vi "Part 2.vi"() -> ()   [LabVIEW 2021]
uses:
  <userlib>/_OpenG.lib/string/string.llb/Convert EOLs (String)__ogtk.vi
  <vilib>/Analysis/NI_AAL_Geometry.lvlib
  <vilib>/Analysis/NI_AALBase.lvlib
  <resource>/lvanlys.dll
  <vilib>/Analysis/baseanly.llb/Real Dot Product.vi
panel:
  out "size(s)":i32=6405262
  in  "Input":string="R 9 (#521d52)\nU 5 (#11e893)\nR 4 (#079312)\nU 4 (#5458e3)\nR 7 (#233422)\nU 3 (#664171)\nL 3 (#475012)\nU 6 (#312e21)\nR 6 (#024a22)\nU 3 (#335f61)\nL 6 (#699da2)\nU 4 (#3d7d41)\nL 6 (#699da0)\nU 7 (#125e51)\nL 3 (#1861e2)\nD 7 (#09f8e1)\nL 4 (#70eb32)\nD 10 (#31c8a3)\nR 4 (#0685e2)\nD 3 (#247e93)\nL 8 (#260972)\nU 7 (#36eca3)\nL 8 (#40b8d2)\nU 5 (#312e23)\nL 7 (#3c4242)\nU 8 (#50c7a3)\nR 6 (#21b062)\nU 7 (#443963)\nL 6 (#0f6920)\nU 5 (#2e1d73)\nL 3 (#6f8330)\nD 3 (#1a4943)\nL 5 (#5cebe2)\nD 12 (#27c9f3)\nR 5 (#220072)\nD 3 (#5adb73)\nL 6 (#317f72)\nD 2 (#053831)\nL 7 (#0c0802)\nU 5 (#124b51)\nL 5 (#198d90)\nD 11 (#46f3b1)\nL 5 (#198d92)\nD 2 (#5424f1)\nL 3 (#1232f2)\nU 4 (#408801)\nL 6 (#18cc52)\nU 4 (#3a6ed1)\nR 6 (#38c312)\nU 5 (#299193)\nL 3 (#2c9e72)\nU 3 (#5c2593)\nR 3 (#2cf822)\nU 5 (#33d851)\nR 4 (#1b0740)\nU 2 (#109221)\nR 9 (#1b0742)\nU 4 (#414cb1)\nL 7 (#0838d2)\nU 5 (#1ea173)\nL 2 (#3fcef2)\nU 7 (#3502f3)\nL 3 (#6d0672)\nU 3 (#0ea733)\nL 4 (#2c94c2)\nU 12 (#4ec103)\nL 4 (#041640)\nD 3 (#4bae23)\nL 3 (#4ff660)\nD 9 (#4bae21)\nL 4 (#458e90)\nD 7 (#202933)\nL 3 (#3fcef0)\nD 6 (#4b45b3)\nR 7 (#710a62)\nD 4 (#111783)\nR 4 (#264f12)\nD 4 (#19e183)\nL 5 (#361fa2)\nD 7 (#19e181)\nL 6 (#27a082)\nD 6 (#188573)\nL 7 (#187f60)\nU 8 (#343903)\nL 4 (#4719a0)\nU 4 (#1abc03)\nL 4 (#0e8d22)\nU 8 (#31faf3)\nL 3 (#7a8270)\nD 12 (#21cf23)\nL 4 (#7a8272)\nD 12 (#2cc503)\nR 4 (#0e8d20)\nD 5 (#0623c3)\nL 9 (#42cc80)\nU 3 (#320273)\nL 2 (#372482)\nU 5 (#11b943)\nL 7 (#10cb12)\nU 10 (#11b941)\nL 2 (#41f692)\nU 5 (#20ece3)\nL 5 (#13b450)\nU 6 (#367f33)\nL 3 (#2a3b50)\nD 9 (#1c7473)\nL 4 (#461d20)\nD 9 (#52f3a1)\nR 4 (#0bc750)\nD 5 (#208061)\nL 6 (#34c310)\nD 2 (#058993)\nL 5 (#0a5680)\nD 6 (#0a6a63)\nL 10 (#1056f0)\nD 2 (#47eba3)\nL 5 (#1056f2)\nD 3 (#3bd443)\nL 7 (#20ad20)\nD 9 (#05bb21)\nL 2 (#1efac0)\nD 7 (#770991)\nL 7 (#429760)\nD 11 (#16ef21)\nL 2 (#365170)\nU 11 (#208063)\nL 8 (#77b350)\nU 6 (#4828a3)\nL 5 (#023210)\nU 5 (#23f413)\nL 3 (#45da92)\nU 4 (#3712a3)\nR 6 (#45da90)\nD 5 (#4805f3)\nR 3 (#1d94d0)\nU 5 (#135023)\nR 5 (#12ee60)\nU 7 (#1ed111)\nL 4 (#1b3730)\nU 11 (#6b41c1)\nL 5 (#3ecd30)\nD 11 (#27e453)\nL 5 (#0e45d2)\nU 3 (#35a2b3)\nL 3 (#0e45d0)\nD 6 (#2c8bd3)\nL 3 (#510880)\nD 8 (#5860e3)\nL 5 (#318662)\nU 5 (#755013)\nL 3 (#318660)\nU 8 (#6ac523)\nL 3 (#233450)\nU 3 (#6aa731)\nL 4 (#498890)\nU 11 (#6aa733)\nR 2 (#46f1c0)\nU 10 (#41ea11)\nR 8 (#22c9f2)\nU 6 (#3198b1)\nR 6 (#7541d0)\nU 7 (#28ad81)\nR 6 (#7541d2)\nD 5 (#295961)\nR 9 (#22c9f0)\nU 5 (#396ab1)\nR 4 (#32ead0)\nU 8 (#4cd1e1)\nR 7 (#372ca0)\nU 5 (#192443)\nL 7 (#0df120)\nU 9 (#3417c3)\nL 5 (#2818d0)\nU 4 (#421ca1)\nR 6 (#444470)\nU 5 (#421ca3)\nL 9 (#147140)\nU 5 (#2c7e73)\nR 9 (#2c5cf0)\nU 3 (#6b8981)\nR 6 (#216860)\nU 6 (#37e4d1)\nR 4 (#10dd20)\nU 8 (#0f9fe1)\nR 3 (#596772)\nU 3 (#52ae11)\nR 7 (#596770)\nU 5 (#1cee91)\nR 4 (#3b6fc0)\nU 7 (#1dcb51)\nL 3 (#2360d0)\nU 4 (#643831)\nL 12 (#4537b0)\nU 4 (#180df1)\nR 9 (#31cd00)\nU 7 (#23f461)\nR 6 (#609520)\nU 7 (#10d611)\nR 3 (#2b2910)\nD 12 (#150921)\nR 5 (#45e700)\nD 5 (#4e7701)\nR 5 (#1eaa20)\nU 7 (#43e531)\nR 9 (#0f10f0)\nU 3 (#29c2d1)\nR 8 (#6ca0d0)\nU 10 (#28c611)\nR 3 (#19ef80)\nD 5 (#4d5381)\nR 9 (#30dd00)\nD 2 (#4c2151)\nR 4 (#480fe0)\nD 5 (#4bdcd1)\nR 4 (#4cc442)\nD 2 (#1122d1)\nR 3 (#08cce2)\nD 6 (#5309a1)\nR 4 (#1118f0)\nD 3 (#1e9b31)\nR 4 (#447830)\nD 10 (#0b6561)\nR 4 (#246dd0)\nD 7 (#5ca761)\nR 5 (#356150)\nD 4 (#09fb01)\nR 6 (#3786e2)\nD 7 (#5f9be1)\nR 7 (#42ca92)\nU 5 (#019611)\nR 8 (#1005b2)\nU 3 (#21ae81)\nR 6 (#173bf2)\nU 4 (#49b611)\nR 3 (#2022c0)\nU 6 (#33a5e1)\nR 8 (#3040d0)\nU 9 (#34b873)\nL 3 (#4a8800)\nU 2 (#34b871)\nL 5 (#06a780)\nU 5 (#08d321)\nL 4 (#4c2b40)\nU 6 (#696b43)\nL 4 (#1ca7c0)\nD 9 (#454c43)\nL 2 (#1f13f0)\nD 2 (#078593)\nL 7 (#1135a0)\nU 9 (#0641a3)\nR 3 (#0bf850)\nU 10 (#6b57e3)\nR 3 (#2d9de2)\nU 4 (#5f4661)\nR 7 (#33d1f2)\nU 6 (#5f4663)\nR 5 (#5a9aa2)\nU 6 (#4fc703)\nR 2 (#4f6cf0)\nU 2 (#0b8203)\nR 11 (#3efc40)\nU 5 (#0b8201)\nR 12 (#2da140)\nU 7 (#20f823)\nR 2 (#380710)\nU 6 (#339af3)\nR 3 (#514cf0)\nD 11 (#087ee3)\nR 7 (#4ad610)\nU 11 (#0e30f1)\nR 7 (#1235d2)\nU 9 (#60a251)\nL 6 (#3c6422)\nU 5 (#60a253)\nL 8 (#33f7d2)\nD 6 (#35e7b1)\nL 6 (#511ed2)\nU 6 (#087321)\nL 5 (#2e2a40)\nU 6 (#38d611)\nR 7 (#233f70)\nU 4 (#143ab1)\nL 10 (#05c470)\nU 4 (#007f61)\nL 5 (#189c70)\nU 4 (#633781)\nR 6 (#568f40)\nU 4 (#258a01)\nR 4 (#0d56c0)\nD 4 (#4866e1)\nR 5 (#4b3420)\nU 3 (#060511)\nR 5 (#100980)\nD 10 (#636631)\nR 2 (#230f20)\nD 3 (#1720b1)\nR 4 (#160300)\nD 2 (#3075f3)\nR 4 (#773320)\nU 2 (#370a93)\nR 3 (#6201c0)\nU 11 (#130763)\nR 8 (#24c420)\nD 9 (#130761)\nR 4 (#4767f0)\nD 4 (#49bd53)\nR 5 (#183ae2)\nD 6 (#36b133)\nL 5 (#6b61f2)\nD 7 (#36b131)\nL 4 (#2a6482)\nD 7 (#4570b3)\nR 6 (#202c82)\nD 4 (#30c3c3)\nR 7 (#2fc410)\nD 8 (#11c203)\nL 8 (#320302)\nD 6 (#1b7b81)\nL 3 (#3abe32)\nD 5 (#1b7b83)\nR 6 (#3a3602)\nU 4 (#05b423)\nR 4 (#598dc0)\nD 4 (#65c873)\nR 3 (#289290)\nD 4 (#188db3)\nL 13 (#2d4af0)\nD 5 (#6ee023)\nR 5 (#3397f0)\nD 3 (#0da5b1)\nR 4 (#1609e0)\nD 4 (#41bb51)\nR 6 (#1609e2)\nD 6 (#380cd1)\nL 6 (#258f60)\nD 5 (#216c73)\nR 2 (#064860)\nD 6 (#207401)\nR 9 (#32e360)\nU 3 (#6788e1)\nR 3 (#47de70)\nD 6 (#74c7a1)\nR 4 (#3b9830)\nD 6 (#05b631)\nL 4 (#5ab730)\nD 3 (#24c2a1)\nR 7 (#090620)\nU 3 (#3e5ff1)\nR 10 (#090622)\nU 7 (#608001)\nL 10 (#150b40)\nU 5 (#1720b3)\nR 6 (#44c360)\nU 8 (#2da851)\nR 6 (#1d1a12)\nU 2 (#21ae41)\nR 2 (#1f8822)\nU 10 (#2d6d01)\nL 3 (#4d4f22)\nU 3 (#2d6d03)\nL 12 (#2c7712)\nU 5 (#21ae43)\nL 9 (#20c892)\nU 7 (#673681)\nR 9 (#0c0af0)\nU 3 (#2a40e1)\nR 4 (#28f0f0)\nU 6 (#5e5341)\nL 5 (#297c60)\nU 5 (#42a051)\nL 9 (#005880)\nU 6 (#538613)\nR 6 (#61c700)\nU 5 (#4d6d83)\nR 8 (#0182a0)\nU 10 (#2a40e3)\nR 5 (#151690)\nU 3 (#4d7ec1)\nR 3 (#69ded0)\nU 7 (#0b8c11)\nR 4 (#13bee0)\nU 2 (#322da1)\nR 5 (#5c33e0)\nU 4 (#3a9c31)\nR 9 (#0736e0)\nD 4 (#1b39f1)\nR 5 (#74b5d0)\nU 8 (#1b39f3)\nR 6 (#02c790)\nU 10 (#3a9c33)\nR 8 (#40c600)\nD 3 (#29d881)\nR 4 (#161380)\nD 11 (#1c3d61)\nL 4 (#6504e0)\nD 3 (#2b9b31)\nR 6 (#1027c0)\nD 5 (#07c691)\nR 5 (#311262)\nD 4 (#469be1)\nL 6 (#0a5bd2)\nD 6 (#2f4b21)\nL 6 (#322842)\nU 6 (#10e413)\nL 5 (#2a9462)\nD 7 (#10e411)\nL 3 (#2f7a02)\nD 6 (#235971)\nR 4 (#448cf0)\nD 6 (#5bc301)\nR 7 (#210c00)\nU 6 (#5bc303)\nR 5 (#2b19f0)\nD 3 (#356581)\nR 4 (#05df90)\nD 7 (#266a01)\nL 11 (#276a82)\nD 5 (#5db6f1)\nR 11 (#4fbb22)\nD 8 (#0025a1)\nR 6 (#69d482)\nU 7 (#409023)\nR 8 (#505ec2)\nU 2 (#1d4c73)\nR 6 (#1c0e12)\nD 7 (#495463)\nR 4 (#534350)\nD 9 (#2a6303)\nL 10 (#3d5a02)\nD 4 (#507ae3)\nR 10 (#3d5a00)\nD 7 (#2d06a3)\nR 7 (#534352)\nD 3 (#03d713)\nR 8 (#3c33d2)\nD 7 (#5bfcf1)\nR 3 (#08c0b0)\nD 2 (#3008b1)\nR 8 (#08c0b2)\nD 4 (#737891)\nR 10 (#05e2d2)\nD 3 (#19a591)\nR 2 (#7106d0)\nD 4 (#332231)\nR 11 (#1d8ae2)\nU 3 (#315711)\nL 8 (#1d8ae0)\nU 4 (#60da61)\nL 2 (#5792c2)\nU 7 (#2095a1)\nL 7 (#197412)\nU 3 (#446241)\nL 6 (#501ba2)\nU 3 (#2b8793)\nL 3 (#2608a2)\nU 3 (#3a64c3)\nL 7 (#3d0f52)\nU 7 (#32efc3)\nL 4 (#447680)\nU 8 (#02e313)\nL 8 (#300890)\nU 8 (#4e0d13)\nR 5 (#0ec4c2)\nU 5 (#3a07f3)\nR 7 (#65ba52)\nU 5 (#201cf3)\nR 4 (#240b72)\nD 2 (#1bb531)\nR 6 (#612f22)\nD 5 (#4c28c1)\nL 4 (#22aaa2)\nD 8 (#3d7bc1)\nR 4 (#23b082)\nD 3 (#379b31)\nR 6 (#05e9e2)\nU 6 (#50a231)\nR 6 (#579442)\nU 3 (#50a233)\nL 6 (#1f1e42)\nU 7 (#379b33)\nR 4 (#1c99e2)\nU 2 (#20b9a1)\nR 7 (#3930c2)\nD 10 (#20b9a3)\nR 6 (#2827d2)\nU 7 (#2ee6f3)\nR 8 (#0c2ce2)\nU 3 (#43d703)\nR 3 (#34aec2)\nD 6 (#67c623)\nR 7 (#547012)\nD 12 (#032bf3)\nR 6 (#15b572)\nU 6 (#6af211)\nR 5 (#1ab422)\nD 6 (#476e93)\nR 9 (#137720)\nD 3 (#4279f3)\nR 4 (#1b0340)\nD 5 (#0e8663)\nL 8 (#74b070)\nD 5 (#0e8661)\nL 7 (#1de0e0)\nU 5 (#40a043)\nL 11 (#157592)\nD 2 (#2cbc01)\nL 6 (#1b5c72)\nD 3 (#04f753)\nR 4 (#615d92)\nD 5 (#04f751)\nR 13 (#16ea52)\nD 6 (#2cbc03)\nR 2 (#0f35b2)\nD 4 (#25a423)\nR 6 (#08bc22)\nD 6 (#603e43)\nR 7 (#4a5c22)\nD 10 (#507d21)\nR 7 (#6ba9b2)\nD 5 (#339b41)\nR 6 (#3603a2)\nD 5 (#416521)\nR 7 (#70c302)\nD 4 (#429121)\nL 4 (#477db2)\nD 5 (#117f11)\nR 10 (#249022)\nU 7 (#657d71)\nR 4 (#15b612)\nU 5 (#19b8e1)\nL 5 (#0d01e0)\nU 8 (#16b691)\nL 3 (#0d8a40)\nU 7 (#3022e1)\nR 8 (#55e320)\nU 10 (#0889d1)\nR 3 (#2e9000)\nU 6 (#49e261)\nR 4 (#0cbee0)\nU 4 (#1aa031)\nR 11 (#5fadc0)\nU 3 (#482851)\nR 2 (#22d1c2)\nU 4 (#2963b1)\nR 5 (#4681b2)\nU 7 (#47e8f1)\nL 6 (#1e3ff2)\nU 6 (#32f5f1)\nR 6 (#2fae52)\nU 3 (#7558d3)\nR 7 (#32c562)\nU 4 (#2ee9c3)\nR 6 (#2164d2)\nU 6 (#19cf81)\nR 4 (#6fbd62)\nD 3 (#35b691)\nR 9 (#3b0f00)\nD 5 (#1fe071)\nR 5 (#3cee10)\nD 5 (#3f7791)\nR 8 (#534340)\nD 4 (#3fb661)\nR 10 (#37c480)\nD 5 (#3fb663)\nR 2 (#6e47a0)\nD 11 (#033cc1)\nR 5 (#1f6410)\nD 6 (#0c70c1)\nL 7 (#0dd340)\nD 7 (#741ab1)\nL 5 (#0dd342)\nD 2 (#1a4621)\nL 7 (#315b10)\nD 6 (#36fbf1)\nL 8 (#58de52)\nD 8 (#42e691)\nL 3 (#58de50)\nD 3 (#08a3a1)\nR 6 (#357dd2)\nD 11 (#3d3941)\nR 5 (#455972)\nD 4 (#349ef1)\nR 8 (#07fd62)\nD 9 (#411051)\nR 6 (#582752)\nU 5 (#4ea411)\nR 3 (#1877c2)\nU 6 (#43e381)\nL 5 (#1877c0)\nU 5 (#26f251)\nR 5 (#34c742)\nU 10 (#50def3)\nR 3 (#0dab82)\nD 3 (#452e53)\nR 6 (#0dab80)\nD 4 (#236ca3)\nR 2 (#31ad52)\nD 3 (#5aab63)\nL 5 (#323322)\nD 10 (#1b03e3)\nR 5 (#4e67f2)\nD 6 (#092371)\nR 7 (#59a6c2)\nD 9 (#246113)\nR 4 (#262360)\nD 10 (#2143d3)\nL 8 (#3b1ce0)\nD 6 (#4de153)\nL 3 (#614042)\nD 8 (#346a63)\nL 8 (#32eec2)\nD 2 (#0a2f53)\nL 6 (#59ea12)\nD 2 (#3a25b1)\nL 6 (#42f560)\nD 8 (#6754a1)\nL 9 (#42f562)\nD 3 (#30a591)\nR 7 (#3f48b2)\nD 4 (#1d40b1)\nR 5 (#25e7c0)\nD 6 (#3e3901)\nR 8 (#25e7c2)\nU 10 (#545bd1)\nR 6 (#2855e2)\nD 11 (#161fa3)\nR 2 (#205752)\nD 5 (#0d60b3)\nL 3 (#1c5862)\nD 4 (#1e2c13)\nL 3 (#6292f2)\nD 7 (#253ac3)\nL 12 (#248f32)\nU 7 (#169ac3)\nL 7 (#018cf2)\nU 4 (#676241)\nL 3 (#043c52)\nD 11 (#161fa1)\nL 7 (#213b42)\nD 4 (#6d64e3)\nL 3 (#17acb0)\nD 6 (#212c53)\nL 4 (#674250)\nU 7 (#1551b3)\nL 12 (#7844a0)\nD 4 (#102593)\nL 2 (#70e432)\nD 3 (#3aa293)\nL 12 (#0ae382)\nD 6 (#277373)\nL 3 (#0e6692)\nU 6 (#5dd281)\nL 9 (#3f08d2)\nU 5 (#5dd283)\nL 2 (#2dfc92)\nU 3 (#3b1ad3)\nR 8 (#4b6390)\nU 10 (#422803)\nR 5 (#052de0)\nU 11 (#2f4123)\nL 6 (#59f040)\nU 3 (#4a9083)\nL 7 (#5b2a40)\nU 8 (#47b583)\nL 3 (#1a0f80)\nU 7 (#11d443)\nL 12 (#27b3c0)\nD 7 (#3cc073)\nL 6 (#63f0f0)\nD 3 (#2cca23)\nL 2 (#33cdb0)\nD 6 (#698a91)\nL 6 (#192830)\nD 4 (#588053)\nL 4 (#1946b0)\nD 6 (#5bf323)\nL 9 (#446402)\nD 7 (#1c7983)\nL 3 (#204152)\nD 8 (#0d93d3)\nL 5 (#3924d2)\nD 4 (#252e03)\nL 7 (#010c80)\nD 7 (#237943)\nL 9 (#010c82)\nD 4 (#33cf23)\nL 2 (#232b42)\nD 5 (#0a8cd1)\nR 4 (#627662)\nD 5 (#45a161)\nL 4 (#124a32)\nD 6 (#1d8e01)\nL 5 (#74c090)\nU 7 (#34ec01)\nL 5 (#36d532)\nU 4 (#03db81)\nR 5 (#6f5072)\nU 8 (#120e73)\nL 3 (#126e52)\nU 3 (#402c63)\nL 5 (#66ec72)\nU 7 (#1d1b63)\nL 3 (#3126f2)\nU 5 (#50e573)\nL 8 (#06c0e2)\nU 5 (#3833d3)\nL 3 (#13e8f2)\nU 6 (#59d571)\nL 4 (#478512)\nD 10 (#59d573)\nL 5 (#3ec962)\nU 10 (#255c03)\nL 5 (#08a472)\nU 6 (#5d8fd1)\nL 4 (#14c112)\nU 7 (#5f4443)\nL 4 (#293aa0)\nU 7 (#1aed53)\nL 2 (#311680)\nU 3 (#63fcc3)\nL 12 (#12d6a2)\nU 5 (#46b3c3)\nL 10 (#12d6a0)\nU 3 (#26d8f3)\nL 10 (#672d90)\nU 9 (#1f2ab3)\nR 8 (#517c62)\nU 10 (#68a6e3)\nL 8 (#2a9692)\nU 5 (#68a6e1)\nL 5 (#456bc2)\nD 4 (#142573)\nL 9 (#0a4712)\nD 7 (#0897f3)\nR 9 (#63e272)\nD 3 (#593dc3)\nL 4 (#63e270)\nD 10 (#415d53)\nL 6 (#459d72)\nD 5 (#1fbed3)\nL 8 (#49c7c2)\nD 4 (#09f433)\nL 2 (#742322)\nD 10 (#02b5c3)\nL 9 (#071b42)\nD 5 (#524e93)\nL 3 (#15a932)\nD 3 (#016c73)\nL 7 (#361b70)\nD 9 (#22a6a1)\nL 3 (#2f8ee0)\nD 7 (#22a6a3)\nL 2 (#2b3d40)\nD 4 (#4df853)\nL 7 (#45ff02)\nD 6 (#26fe93)\nL 10 (#5a0862)\nD 7 (#2d1e83)\nL 5 (#06e520)\nD 6 (#2410d3)\nL 9 (#1b49e0)\nD 2 (#46d233)\nL 7 (#32b7f0)\nD 8 (#67f703)\nL 5 (#296ba0)\nU 7 (#67f701)\nL 7 (#367c00)\nU 5 (#46d231)\nR 7 (#359260)\nU 3 (#2e68b3)\nL 4 (#450ba0)\nU 2 (#2f88f3)\nL 8 (#3ca9e2)\nD 7 (#1631d3)\nL 6 (#770e30)\nD 10 (#47c983)\nL 5 (#770e32)\nU 5 (#260fc3)\nL 12 (#3ca9e0)\nU 6 (#1ee513)\nR 12 (#75c272)\nU 3 (#0aadf3)\nL 2 (#0272a2)\nU 7 (#4ebd23)"
  in  "Example":string="R 6 (#70c710)\nD 5 (#0dc571)\nL 2 (#5713f0)\nD 2 (#d2c081)\nR 2 (#59c680)\nD 2 (#411b91)\nL 5 (#8ceee2)\nU 2 (#caa173)\nL 1 (#1b58a2)\nU 2 (#caa171)\nR 2 (#7807d2)\nU 3 (#a77fa3)\nL 2 (#015232)\nU 2 (#7a21e3)"
  out "Output":i64=952408144115
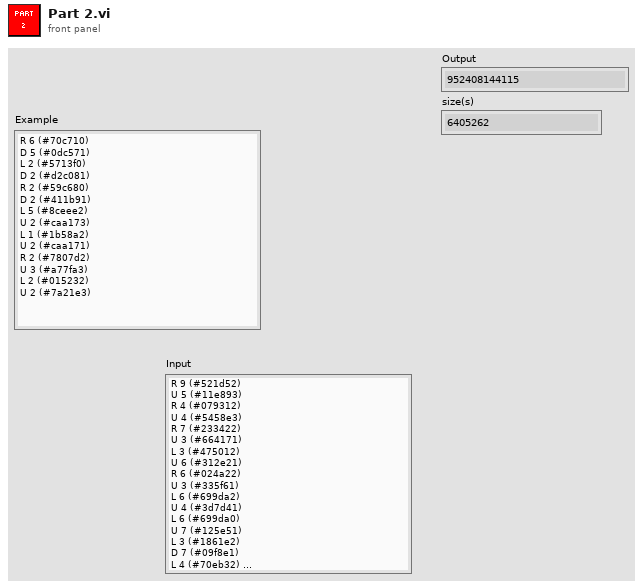
[diagram p1: front panel]
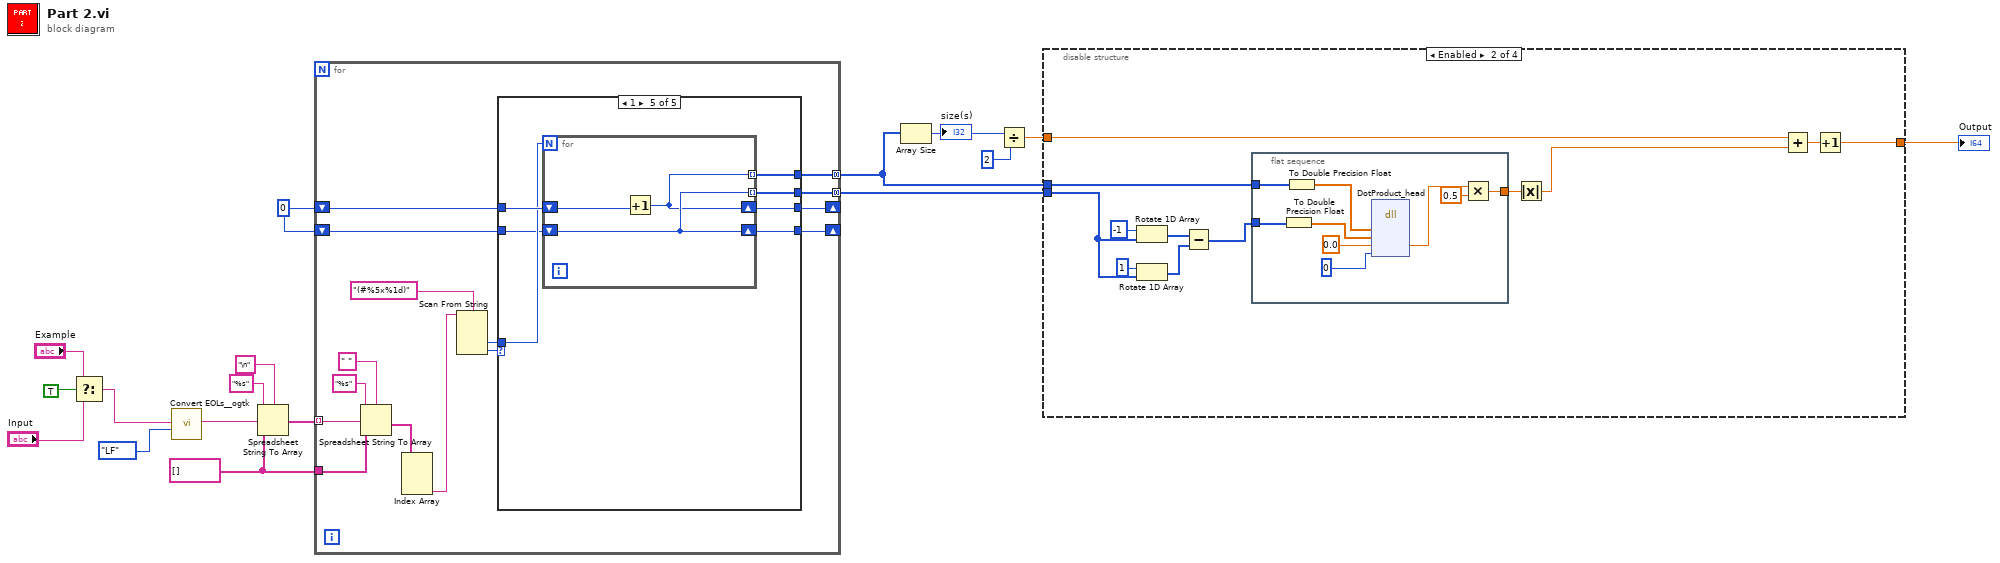
[diagram p0: block diagram]
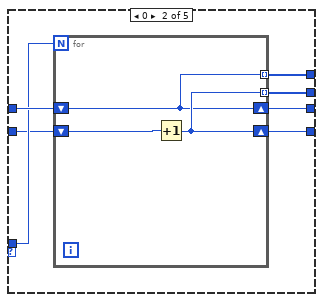
[diagram p3: hidden frame]
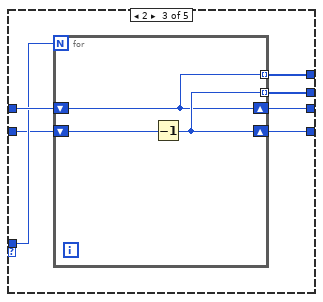
[diagram p4: hidden frame]
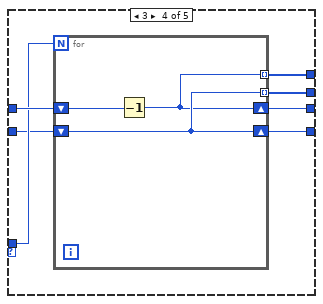
[diagram p5: hidden frame]
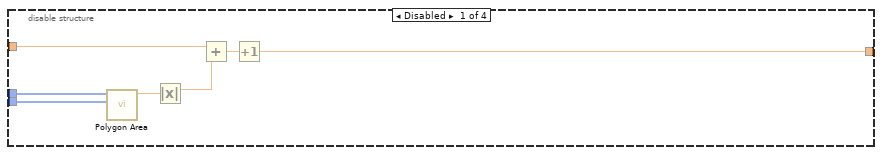
[diagram p6: hidden frame]
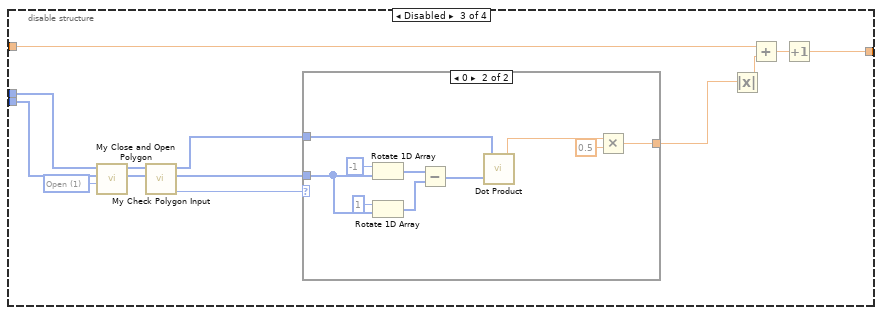
[diagram p7: hidden frame]
diagram:
  w9 = 0
  w12 = string[] []
  n1 = Select(t="Example", s=TRUE, f="Input") -> (s? t:f=w5:string)
  n2 = call-poly <userlib>:"Convert EOLs__ogtk.vi"("Convert to:"=enum16{"CR", "LF", "CRLF"}."LF", "String in"=w5) -> ("String out"=w15:string)  [unwired: 9 in]
  n3 = Spreadsheet String To Array(delimiter (Tab)="\n", format string="%s", spreadsheet string=w15, array type (2D Dbl)=w12) -> (array=w13:string[])
  n4 = for {
    tunnel: w13 -> [w31] mode=indexing
    tunnel: w12 -> [w30]
    shift-right: [w26] -> _
    shift-left: w9 -> [w27]
    tunnel: [w25] -> w1 mode=concatenating
    shift-right: [w23] -> _
    shift-left: w9 -> [w24]
    tunnel: [w22] -> w2 mode=concatenating
    n5 = Spreadsheet String To Array(delimiter (Tab)=" ", format string="%s", spreadsheet string=w31, array type (2D Dbl)=w30) -> (array=w28:string[])
    n6 = Index Array(array=w28) -> (element #3=w21:string)  [unwired: 3 in, 2 out]
    n7 = Scan From String(format string="(#%5x%1d)", input string=w21) -> (output 1=w18:u32, output 2=w19:i32)  [unwired: 4 in, 3 out]
    n8 = case shown="1" w19 {
      tunnel: w27 -> [w34 w41 w51 w61 w71]
      tunnel: [w34 w40 w50 w60 w70] -> w26
      tunnel: w18 -> [_ w39 w49 w59 w69]
      tunnel: [_ w38 w45 w55 w65] -> w25
      tunnel: w24 -> [w33 w37 w48 w58 w68]
      tunnel: [w33 w36 w47 w57 w67] -> w23
      tunnel: [_ w35 w46 w56 w66] -> w22
      frame Default {
      }
      frame 0 {
        n9 = for {
          N: w39 -> [_]
          shift-right: [w43] -> w40
          shift-left: w41 -> [w43]
          tunnel: [w44] -> w38 mode=indexing
          shift-right: [w44] -> w36
          shift-left: w37 -> [w42]
          tunnel: [w43] -> w35 mode=indexing
          n10 = Increment(x=w42) -> (x+1=w44:i32)
        }
      }
      frame 2 {
        n11 = for {
          N: w49 -> [_]
          shift-right: [w52] -> w50
          shift-left: w51 -> [w52]
          tunnel: [w53] -> w45 mode=indexing
          shift-right: [w53] -> w47
          shift-left: w48 -> [w54]
          tunnel: [w52] -> w46 mode=indexing
          n12 = Decrement(x=w54) -> (x-1=w53:i32)
        }
      }
      frame 3 {
        n13 = for {
          N: w59 -> [_]
          shift-right: [w62] -> w60
          shift-left: w61 -> [w63]
          tunnel: [w64] -> w55 mode=indexing
          shift-right: [w64] -> w57
          shift-left: w58 -> [w64]
          tunnel: [w62] -> w56 mode=indexing
          n14 = Decrement(x=w63) -> (x-1=w62:i32)
        }
      }
      frame 1 {
        n15 = for {
          N: w69 -> [_]
          shift-right: [w72] -> w70
          shift-left: w71 -> [w73]
          tunnel: [w74] -> w65 mode=indexing
          shift-right: [w74] -> w67
          shift-left: w68 -> [w74]
          tunnel: [w72] -> w66 mode=indexing
          n16 = Increment(x=w73) -> (x+1=w72:i32)
        }
      }
    }
  }
  n17 = Array Size(array=w2) -> (size(s)=w11:i32)
  "size(s)" <- w11
  n18 = Divide(x=w11, y=2) -> (x/y=w10:dbl)
  n19 = disable-structure shown="Enabled" {
    disable-tunnel: w10 -> [w79 w93 w115 _]
    disable-tunnel: w2 -> [w76 w89 w105 _]
    disable-tunnel: [w75 w91 w112 _] -> w7
    disable-tunnel: w1 -> [w77 w82 w104 _]
    frame Disabled {
      n20 = call <vilib>:"Polygon Area.vi"("Y"=w77, "X"=w76) -> ("signed area"=w81:dbl)  [unwired: 8 in, 1 out]
      n21 = Absolute Value(x=w81) -> (abs(x)=w80:dbl)
      n22 = Add(x=w79, y=w80) -> (x+y=w78:dbl)
      n23 = Increment(x=w78) -> (x+1=w75:dbl)
    }
    frame Enabled {
      n24 = Rotate 1D Array(1:w82, 2:-1 ("n")) -> (0:w84:i32[])
      n25 = Rotate 1D Array(1:w82, 2:1 ("n")) -> (0:w86:i32[])
      n26 = Subtract(x=w84, y=w86) -> (x-y=w83:i32[])
      n27 = flat-sequence {
        tunnel: [w101] -> w90
        tunnel: w83 -> [w98]
        tunnel: w89 -> [w97]
        frame #0 {
          n28 = To Double Precision Float(number=w98) -> (double precision float=w94:dbl[])
          n29 = To Double Precision Float(number=w97) -> (double precision float=w95:dbl[])
          n30 = dll-call lib="C:/Program Files (x86)/National Instruments/LabVIEW 2021/resource/lvanlys.*" fn="DotProduct_head"("X Vector"=w95, "Y Vector"=w94, 0.0, 0) -> (w96:dbl)  [unwired: 7 in, 2 out]
          n31 = Multiply(x=w96, y=0.5) -> (x*y=w101:dbl)
        }
      }
      n32 = Absolute Value(x=w90) -> (abs(x)=w88:dbl)
      n33 = Add(x=w93, y=w88) -> (x+y=w92:dbl)
      n34 = Increment(x=w92) -> (x+1=w91:dbl)
    }
    frame Disabled {
      w108 = u16 1 items=["Closed", "Open"] ("type")
      n35 = call "My Close and Open Polygon.vi"("type"=w108, "Y In"=w104, "X In"=w105) -> ("Y Out"=w106:i32[], "X Out"=w107:i32[])  [unwired: 7 in]
      n36 = call "My Check Polygon Input.vi"("Y In"=w106, "X In"=w107) -> ("error"=w109:i32, "Y Out"=w111:i32[], "X Out"=w110:i32[])  [unwired: 7 in]
      n37 = case shown="0" w109 {
        tunnel: [_ w119] -> w103
        tunnel: w110 -> [_ w118]
        tunnel: w111 -> [_ w120]
        frame -1, Default {
        }
        frame 0 {
          n38 = Rotate 1D Array(1:w120, 2:-1 ("n")) -> (0:w121:i32[])
          n39 = Rotate 1D Array(1:w120, 2:1 ("n")) -> (0:w123:i32[])
          n40 = Subtract(x=w121, y=w123) -> (x-y=w117:i32[])
          n41 = call-poly <vilib>:"Dot Product.vi"("Y Vector"=w117, "X Vector"=w118) -> ("X * Y"=w116:dbl)  [unwired: 1 out]
          n42 = Multiply(x=w116, y=0.5) -> (x*y=w119:dbl)
        }
      }
      n43 = Absolute Value(x=w103) -> (abs(x)=w113:dbl)
      n44 = Add(x=w115, y=w113) -> (x+y=w114:dbl)
      n45 = Increment(x=w114) -> (x+1=w112:dbl)
    }
    frame Disabled {
    }
  }
  "Output" <- w7
